vi "000 Write Error.vi"(8 "error in (no error)":errorcluster caption="Error In", 9 "Data":variant, 10 "Name":string, 11 "Path":path) -> (0 "error out":errorcluster caption="Error Out", 3 "Error":string)   [LabVIEW 2020]
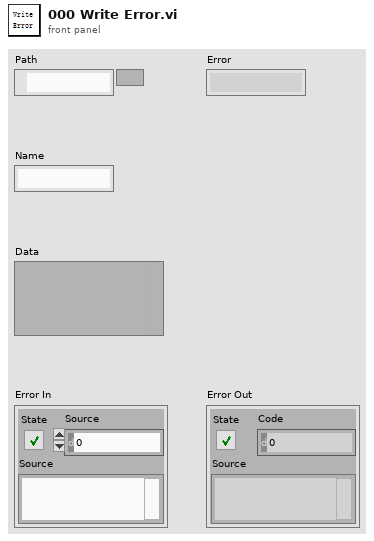
[diagram p1: front panel]
types:
  T1 = cluster{"status":bool, "code":bool, "source":bool}
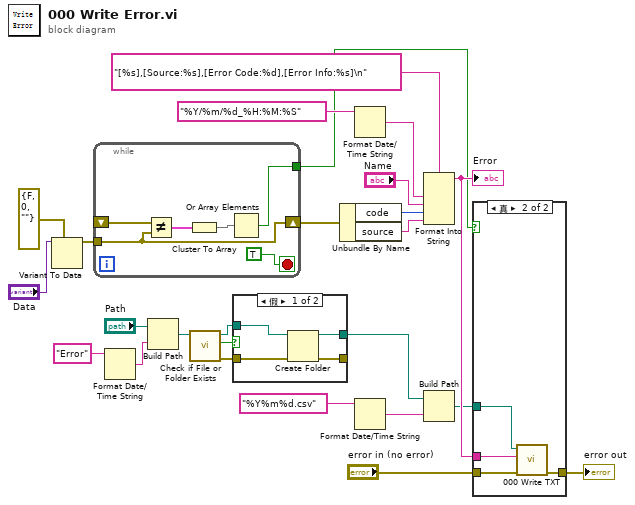
[diagram p0: block diagram]
diagram:
  n1 = Variant To Data(type=errorcluster {"status"=FALSE, "code"=0, "source"=""} ("error in (no error)"), Variant="Data") -> (data=w8:errorcluster)  [unwired: 1 in, 1 out]
  n2 = while {
    tunnel: w8 -> [w30]
    shift-right: [w30] -> w6
    shift-left: _ -> [w31]
    tunnel: [w26] -> w7
    stop <- TRUE stop-if-true
    n3 = Not Equal?(x=w31, y=w30) -> (x != y?=w29:T1)
    n4 = Cluster To Array(cluster=w29) -> (array=w28:bool[])
    n5 = Or Array Elements(Boolean array=w28) -> (logical OR=w26:bool)
  }
  n6 = Format Date/Time String(time format string (%c)="Error" ("时间格式字符串(%c)")) -> (date/time string=w20:string)  [unwired: 2 in]
  n7 = Build Path(base path="Path", name or relative path=w20) -> (appended path=w19:path)
  n8 = call <vilib>:"Check if File or Folder Exists.vi"("path"=w19) -> ("error out"=w5:errorcluster, "file or folder exists?"=w3:bool, "dup path"=w4:path)  [unwired: 8 in]
  n9 = case shown="假" w3 {
    tunnel: w4 -> [w35 w36]
    tunnel: w5 -> [w34 w37]
    tunnel: [w33 w37] -> _
    tunnel: [w32 w36] -> w17
    frame False {
      n10 = Create Folder(path (use dialog)=w35, error in=w34) -> (created path=w32:path, error out=w33:errorcluster)  [unwired: 1 in, 1 out]
    }
    frame True {
    }
  }
  n11 = Unbundle By Name(w6) -> ("code"=w24:i32, "source"=w23:string)
  n12 = Format Date/Time String(time format string (%c)="%Y/%m/%d_%H:%M:%S" ("时间格式字符串(%c)")) -> (date/time string=w22:string)  [unwired: 2 in]
  n13 = Format Date/Time String(time format string (%c)="%Y%m%d.csv" ("时间格式字符串(%c)")) -> (date/time string=w1:string)  [unwired: 2 in]
  n14 = Format Into String(format string="[%s],[Source:%s],[Error Code:%d],[Error Info:%s]\n" ("格式字符串"), w22, "Name", w24, w23) -> (resulting string=w18:string)  [unwired: 2 in, 1 out]
  "Error" <- w18
  n15 = Build Path(base path=w17, name or relative path=w1) -> (appended path=w16:path)
  n16 = case shown="真" w7 {
    tunnel: w18 -> [_ w42]
    tunnel: w16 -> [_ w41]
    tunnel: "error in (no error)" -> [w38 w40]
    tunnel: [w38 w39] -> w9
    frame False {
    }
    frame True {
      n17 = call "000 Write TXT.vi"("error in (no error)"=w40, "txt"=w42, "Path"=w41) -> ("error out"=w39:errorcluster)  [unwired: 8 in]
    }
  }
  "error out" <- w9
